vi "Lab_2_mainVI_Ashish.vi"() -> ()   [LabVIEW 2020]
panel:
  out "Steady-state inflow Tank1":dbl
  out "H2":dbl(graph)
  out "H1":dbl(graph)
  in  "hss,2":dbl
  in  "A2":dbl
  in  "A1":dbl
  in  "a2":dbl
  in  "a1":dbl
  in  "U":dbl
  out "Tank 2":dbl(slide) scale=0.0..100.0
  out "Tank 1":dbl(slide) scale=0.0..100.0
  in  "stop":bool
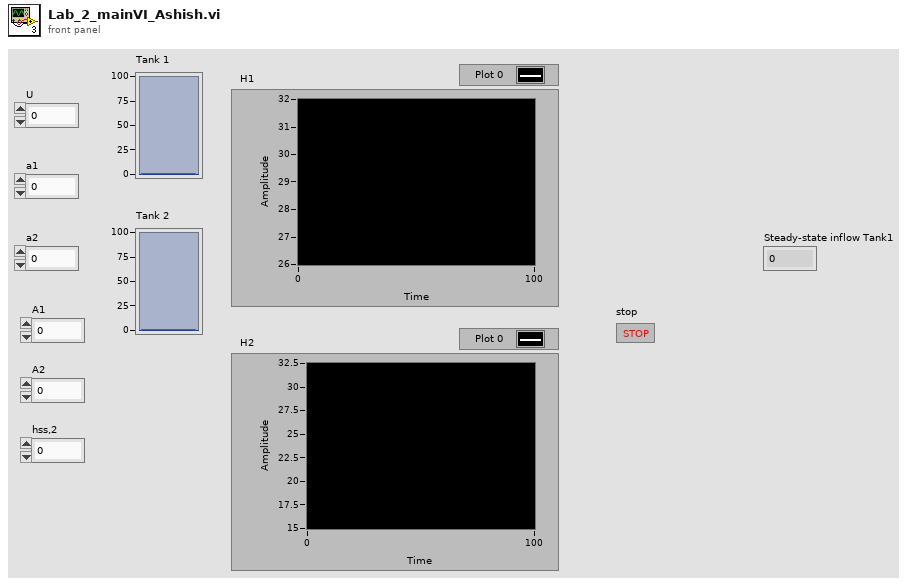
[diagram p1: front panel]
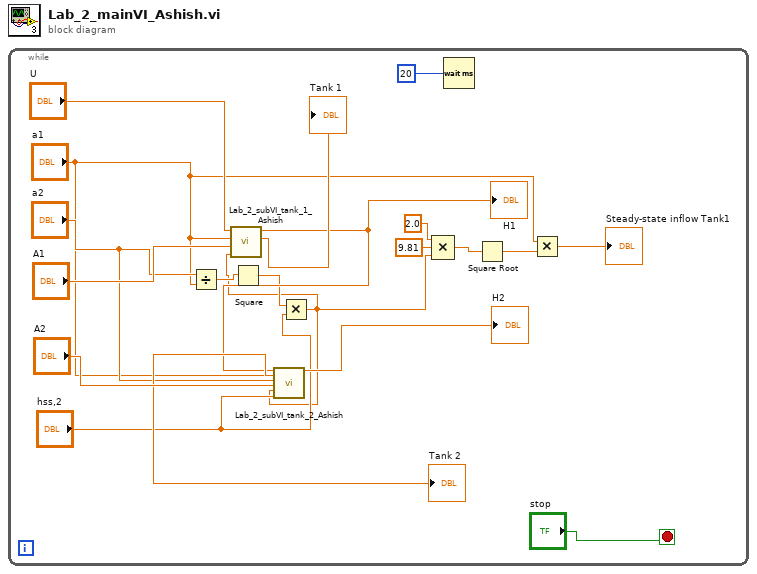
[diagram p0: block diagram]
diagram:
  n1 = while {
    stop <- "stop" stop-if-true
    n2 = Divide(x="a2", y="a1") -> (x/y=w10:dbl)
    n3 = Square(x=w10) -> (x^2=w9:dbl)
    n4 = Multiply(x=w9, y="hss,2") -> (x*y=w2:dbl)
    n5 = call "Lab_2_subVI_tank_1_Ashish.vi"("hss,1"=w2, "A1"="A1", "a1"="a1", "U"="U") -> ("height tank1"=→"Tank 1":dbl, "H1"=w13:dbl)  [unwired: 6 in]
    "H1" <- w13
    n6 = call "Lab_2_subVI_tank_2_Ashish.vi"("H1"=w13, "a1"="a1", "a2"="a2", "A2"="A2", "hss,1"=w2, "hss,2"="hss,2") -> ("H 2"=→"H2":dbl, "h2"=→"Tank 2":dbl)  [unwired: 12 in]
    n7 = Compound Arithmetic op=MULTIPLY(2.0 ("value"), 9.81 ("value"), w2) -> (w5:dbl)
    n8 = Wait (ms)(milliseconds to wait=u32 20 ("millisecond timer value")) -> ()  [unwired: 1 out]
    n9 = Square Root(x=w5) -> (sqrt(x)=w3:dbl)
    n10 = Multiply(x="a1", y=w3) -> (x*y=→"Steady-state inflow Tank1":dbl)
  }
